vi "Mask and Histogram.vi"(0 "ROI Descriptor (Image Mask 1)":T1={"Global Rectangle"=[313, 248, 531, 496], "Contours"=[{"ID"=enum."External", "Type"=3, "Coordinates"=[313, 248, 531, 496]}]} {"Contours"."Type" items=["No Selection", "Point", "Line", "Rectangle", "Oval", "Polygon", "Freehand Region", "Annulus", "Unused2", "Unused3", "Broken Line", "Freehand Line", "Rotated Rectangle"]}, 1 "Out / In (Image Mask 1)":bool, 2 "ROI Descriptor (Histogram 1)":T1 {"Contours"."Type" items=["No Selection", "Point", "Line", "Rectangle", "Oval", "Polygon", "Freehand Region", "Annulus", "Unused2", "Unused3", "Broken Line", "Freehand Line", "Rotated Rectangle"]}, 7 "error in":errorcluster) -> (20 "Histogram (Histogram 1)":u32[][](array[numeric]), 21 "Statistics (Histogram 1)":T3 {"Standard  Variation" format="%.2f"; "Mean Value" format="%.2f"; "Maximal Value" format="%.2f"; "Minimal Value" format="%.2f"}, 27 "error out":errorcluster)   [LabVIEW 2014]
panel:
  out "Image Out":T2(plugin-control)
  out "Histogram Graph":u32[][](graph)
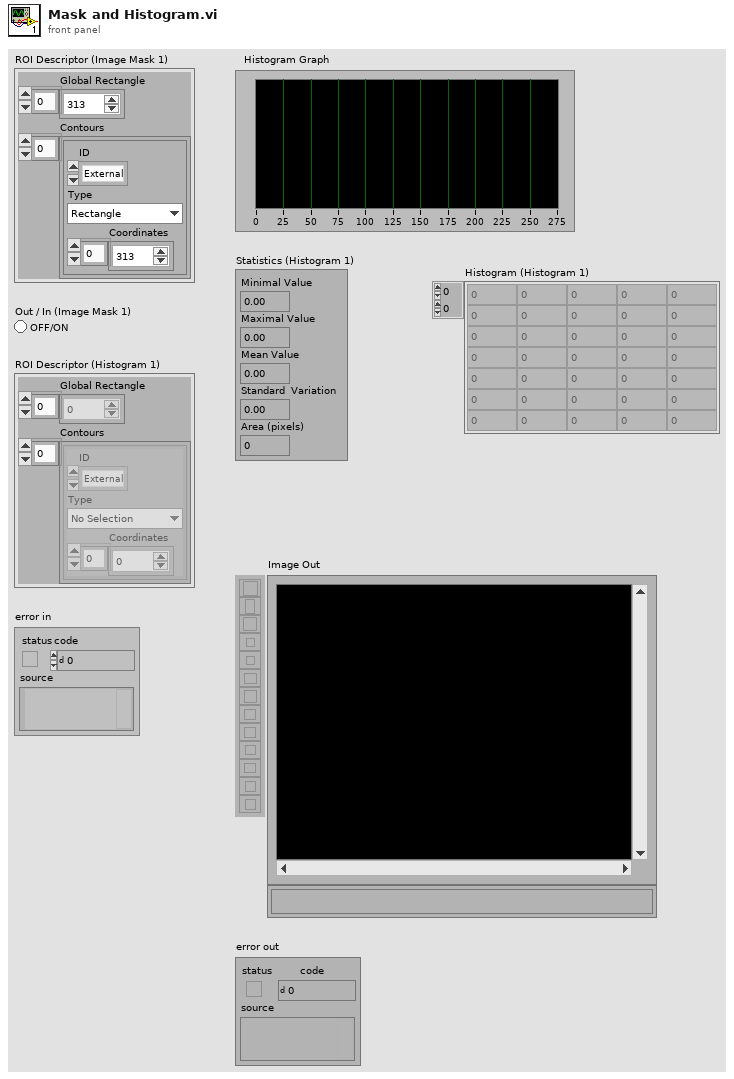
[diagram p1: front panel]
types:
  T1 = cluster{"Global Rectangle":i32[], "Contours":cluster{"ID":enum32{"External", "Internal"}, "Type":u32, "Coordinates":i32[]}[]}
  T2 = typedef "IMAQ Image.ctl" = refnum<image>
  T3 = cluster{"Minimal Value":sgl, "Maximal Value":sgl, "Mean Value":sgl, "Standard  Variation":sgl, "Area (pixels)":i32}
  T4 = typedef "Image Type" = u32
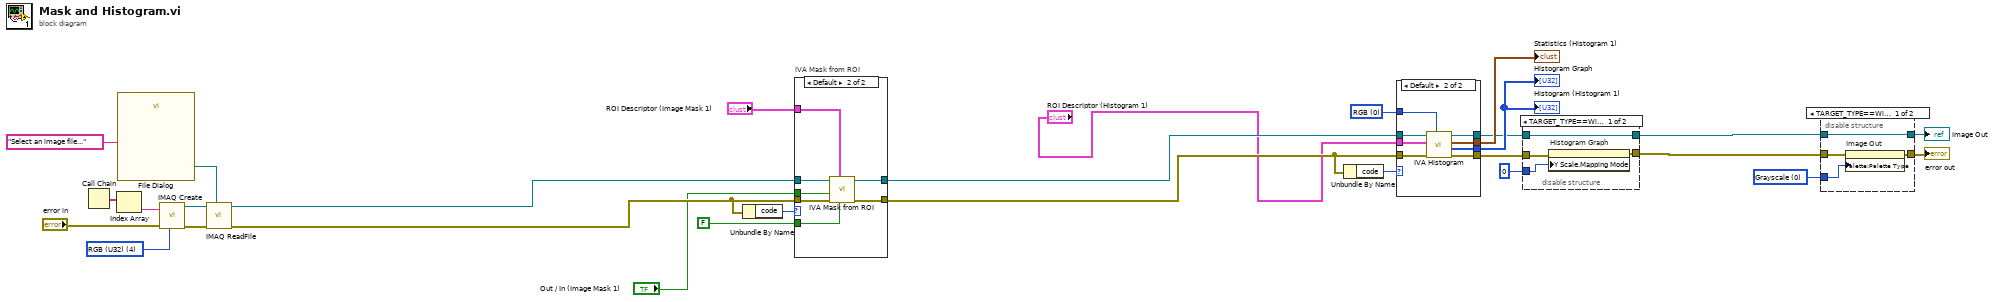
[diagram p0: block diagram]
diagram:
  w1 = u32 0 items=["Grayscale", "Binary", "Gradient", "Rainbow", "Temperature", "User Defined"] ("Palette")
  w11 = u16 0 items=["RGB", "HSL", "HSV", "HSI"] ("Color Mode")
  w21 = T4 4 items=["Grayscale (U8)", "Grayscale (I16)", "Grayscale (SGL)", "Complex (CSG)", "RGB (U32)", "HSL (U32)", "RGB (U64)", "Grayscale (U16)"] ("Image Type")
  n1 = Call Chain() -> (call chain=w25:string[])
  n2 = Index Array(array=w25) -> (element=w24:string)  [unwired: 1 in]
  n3 = call "File Dialog"("prompt"="Select an image file...") -> ("selected path"=w22:path)  [unwired: 6 in, 8 out]
  n4 = call "IMAQ Create"("Image Name"=w24, "Image Type"=w21, "error in (no error)"="error in") -> ("New Image"=w28:T2, "error out"=w27:errorcluster)  [unwired: 1 in, 1 out]
  n5 = call "IMAQ ReadFile"("File Path"=w22, "error in (no error)"=w27, "Image"=w28) -> ("error out"=w29:errorcluster, "Image Out"=w18:T2)  [unwired: 2 in, 5 out]
  n6 = Unbundle By Name(w29) -> ("code"=w15:i32)
  n7 = case "IVA Mask from ROI" shown="Default" w15 {
    tunnel: "ROI Descriptor (Image Mask 1)" -> [_ w37]
    tunnel: FALSE ("Shrink") -> [_ w36]
    tunnel: w18 -> [w30 w35]
    tunnel: w29 -> [_ w34]
    tunnel: [_ w33] -> w17
    tunnel: [w30 w32] -> w14
    tunnel: "Out / In (Image Mask 1)" -> [_ w31]
    frame -1074396199, -1074396198 {
      # "Discard\nCoordinate\nSystem\nError"
    }
    frame Default {
      n8 = call <vilib>:"IVA Mask from ROI.vi"("Shrink"=w36, "ROI Descriptor"=w37, "error in (no error)"=w34, "Out / In"=w31, "Image Src"=w35) -> ("error out"=w33:errorcluster, "Image Out"=w32:T2)  [unwired: 5 out]
    }
  }
  n9 = Unbundle By Name(w17) -> ("code"=w7:i32)
  n10 = case shown="Default" w7 {
    tunnel: w17 -> [_ w46]
    tunnel: w14 -> [w38 w45]
    tunnel: [_ w44] -> w13
    tunnel: [_ w43] -> w12
    tunnel: w11 -> [_ w42]
    tunnel: [_ w41] -> w10
    tunnel: "ROI Descriptor (Histogram 1)" -> [_ w40]
    tunnel: [w38 w39] -> w6
    frame -1074396199, -1074396198 {
      # "Discard\nCoordinate\nSystem\nError"
    }
    frame Default {
      n11 = call <vilib>:"IVA Histogram.vi"("Color Mode"=w42, "error in (no error)"=w46, "ROI Descriptor"=w40, "Image In"=w45) -> ("error out"=w43:errorcluster, "Histograms"=w41:u32[][], "Statistics"=w44:T3, "Image Out"=w39:T2)  [unwired: 4 out]
    }
  }
  "Histogram Graph" <- w10
  "Statistics (Histogram 1)" <- w13
  "Histogram (Histogram 1)" <- w10
  n12 = disable-structure "Conditional Disable Structure" shown="TARGET_TYPE==Windows" {
    disable-tunnel: w12 -> [w50 w51]
    disable-tunnel: [w49 w51] -> w8
    disable-tunnel: w6 -> [w48 w52]
    disable-tunnel: [w48 w52] -> w3
    disable-tunnel: u8 0 ("Y Scale.Mapping Mode") -> [w47 _]
    frame condition #0 (active) {
      n13 = property on="Histogram Graph" class="WFGraph (strict)"(error in=w50, "Y Scale.Mapping Mode"=w47) -> (error out=w49:errorcluster)  [unwired: 1 in, 1 out]
    }
    frame condition #1 {
    }
  }
  n14 = disable-structure "Conditional Disable Structure" shown="TARGET_TYPE==Windows" {
    disable-tunnel: w8 -> [w56 w57]
    disable-tunnel: [w55 w57] -> w4
    disable-tunnel: w3 -> [w54 w58]
    disable-tunnel: [w54 w58] -> w2
    disable-tunnel: w1 -> [w53 _]
    frame condition #0 (active) {
      n15 = property on="Image Out" class="ImageControl"(error in=w56, "Palette:Palette Type"=w53) -> (error out=w55:errorcluster)  [unwired: 1 in, 1 out]
    }
    frame condition #1 {
    }
  }
  "error out" <- w4
  "Image Out" <- w2
